vi "Test Red-y Pressure Control CFG1.vi"(11 "Test Case In":refnum<class "Test Red-y Pressure Control CFG.lvclass">) -> (0 "error out":errorcluster, 3 "Test Case Out":refnum<class "Test Red-y Pressure Control CFG.lvclass">)   [LabVIEW 2024, in "Test Red-y Pressure Control CFG.lvclass"]
uses:
  Test Red-y Pressure Control CFG.lvclass
  C:/Program Files/National Instruments/LabVIEW 2024/vi.lib/Astemes/LUnit/Test Case.lvclass
  MSS/MSS.lvclass
  Strategies/Red-y Read Write/Perform Action Red-y Read Write Strategy.lvclass
  Configurations/Pressure Control CFG/Red-y Pressure Control CFG.lvclass
  Configurations/Pressure Control CFG Simulated/Red-y Pressure Control CFG Simulated.lvclass
  <vilib>/Astemes/LUnit/Test Case.lvclass/Test Case.ctl
  <vilib>/Astemes/LUnit/Append Pass Result.vi
  <vilib>/Astemes/LUnit/Append Fail Result.vi
  <vilib>/Astemes/LUnit/Run In UI.vi
  <vilib>/Utility/error.llb/Clear Errors.vi
  <vilib>/Astemes/LUnit/Test Case.lvclass
panel:
  out "Pressure Scaling Max":variant
  out "Signal Type AI":variant
  out "Pressure":variant
  out "Output":variant
  out "Temperature":variant
  out "Flow":variant
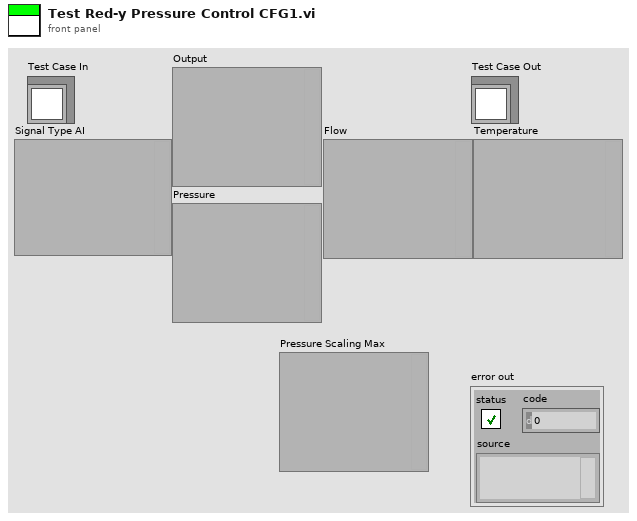
[diagram p1: front panel]
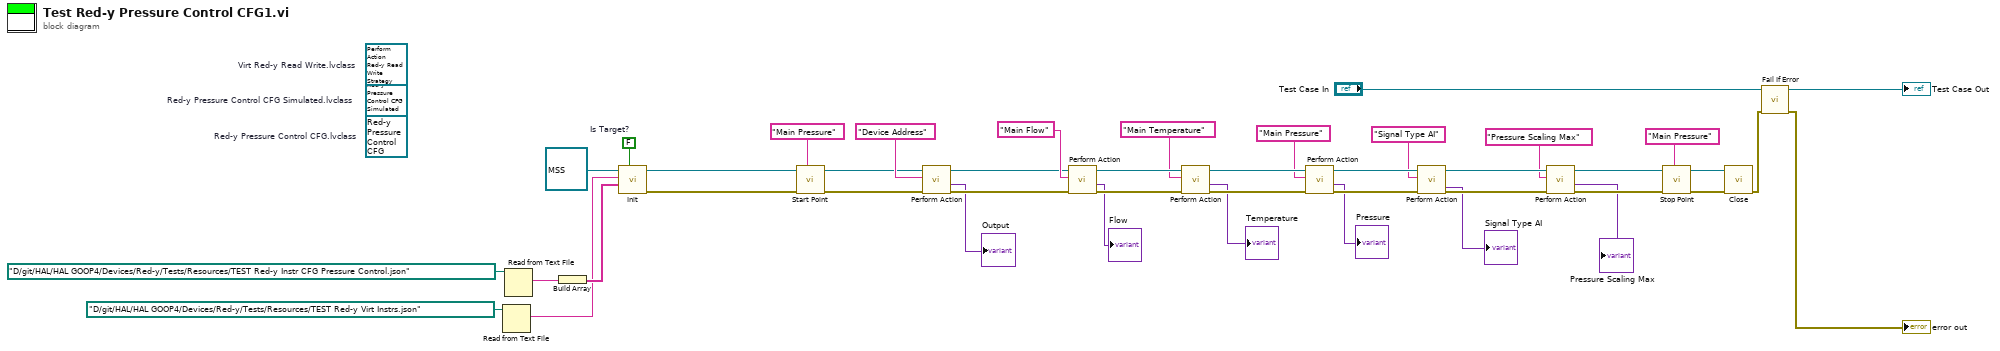
[diagram p0: block diagram]
diagram:
  (unwired) refnum<class "Red-y Pressure Control CFG Simulated.lvclass"> refnum  # Red-y Pressure Control CFG Simulated.lvclass
  (unwired) refnum<class "Red-y Pressure Control CFG.lvclass"> refnum  # Red-y Pressure Control CFG.lvclass
  (unwired) refnum<class "Perform Action Red-y Read Write Strategy.lvclass"> refnum  # Virt Red-y Read Write.lvclass
  w37 = FALSE  # Is Target?
  n1 = Read from Text File(file (use dialog)=path "D:/git/HAL/HAL GOOP4/Devices/Red-y/Tests/Resources/TEST Red-y Virt Instrs.json") -> (text=w1:string)  [unwired: 3 in, 3 out]
  n2 = Read from Text File(file (use dialog)=path "D:/git/HAL/HAL GOOP4/Devices/Red-y/Tests/Resources/TEST Red-y Instr CFG Pressure Control.json") -> (text=w3:string)  [unwired: 3 in, 3 out]
  n3 = Build Array(w3) -> (w36:string[])
  n4 = call "Init.vi"("Is Target?"=w37, "Instr CFGs"=w36, "<JSON> Virt Instr CFG"=w1, "MSS in"=refnum<class "MSS.lvclass"> refnum ("HAL GOOP4.lvlib:Measure and Stimulus Subsystems.lvclass")) -> ("error out"=w39:errorcluster, "MSS out"=w38:refnum<class "MSS.lvclass">)  [unwired: 4 in, 2 out]
  n5 = call "Start Point.vi"("Task-Point Ident"="Main Pressure", "error in"=w39, "MSS in"=w38) -> ("error out"=w21:errorcluster, "MSS out"=w20:refnum<class "MSS.lvclass">)  [unwired: 7 in]
  n6 = call "Perform Action.vi"("error in"=w21, "Point Ident"="Device Address", "MSS in"=w20) -> ("error out"=w28:errorcluster, "Output"=→"Output":variant, "MSS out"=w27:refnum<class "MSS.lvclass">)  [unwired: 5 in, 1 out]
  n7 = call "Perform Action.vi"("error in"=w28, "Point Ident"="Main Flow" ("Task-Point Idents"), "MSS in"=w27) -> ("error out"=w35:errorcluster, "Output"=→"Flow":variant, "MSS out"=w31:refnum<class "MSS.lvclass">)  [unwired: 5 in, 1 out]
  n8 = call "Perform Action.vi"("error in"=w35, "Point Ident"="Main Temperature", "MSS in"=w31) -> ("error out"=w32:errorcluster, "Output"=→"Temperature":variant, "MSS out"=w23:refnum<class "MSS.lvclass">)  [unwired: 5 in, 1 out]
  n9 = call "Perform Action.vi"("error in"=w32, "Point Ident"="Main Pressure", "MSS in"=w23) -> ("error out"=w24:errorcluster, "Output"=→"Pressure":variant, "MSS out"=w13:refnum<class "MSS.lvclass">)  [unwired: 5 in, 1 out]
  n10 = call "Perform Action.vi"("error in"=w24, "Point Ident"="Signal Type AI", "MSS in"=w13) -> ("error out"=w14:errorcluster, "Output"=→"Signal Type AI":variant, "MSS out"=w9:refnum<class "MSS.lvclass">)  [unwired: 5 in, 1 out]
  n11 = call "Perform Action.vi"("error in"=w14, "Point Ident"="Pressure Scaling Max", "MSS in"=w9) -> ("error out"=w10:errorcluster, "Output"=→"Pressure Scaling Max":variant, "MSS out"=w8:refnum<class "MSS.lvclass">)  [unwired: 5 in, 1 out]
  n12 = call "Stop Point.vi"("Task-Point Ident"="Main Pressure" ("Task-Point Idents"), "error in"=w10, "MSS in"=w8) -> ("error out"=w18:errorcluster, "MSS out"=w17:refnum<class "MSS.lvclass">)  [unwired: 7 in]
  n13 = call "Close.vi"("error in"=w18, "MSS in"=w17) -> ("error out"=w5:errorcluster)  [unwired: 8 in, 1 out]
  n14 = call <vilib>:"Fail If Error.vi"("error in (no error)"=w5, "LUnit Test Case In"="Test Case In") -> ("error out"=→"error out":errorcluster, "LUnit Test Case Out"=→"Test Case Out":refnum<class "Test Red-y Pressure Control CFG.lvclass">)  [unwired: 8 in]
